vi "Assign X Coordinate.vi"(7 "Column Gap":i32=30, 10 "Order":T2[](array[typedef]), 11 "Decision Tree Out in":T1) -> (3 "Decision Tree Out out":T1)   [LabVIEW 2025]
uses:
  Types/Decision Tree.ctl
  Types/Sequencing Tree Node.ctl
  Types/Single Cmd Info.ctl
  <vilib>/picture/picture.llb/imagedata.ctl
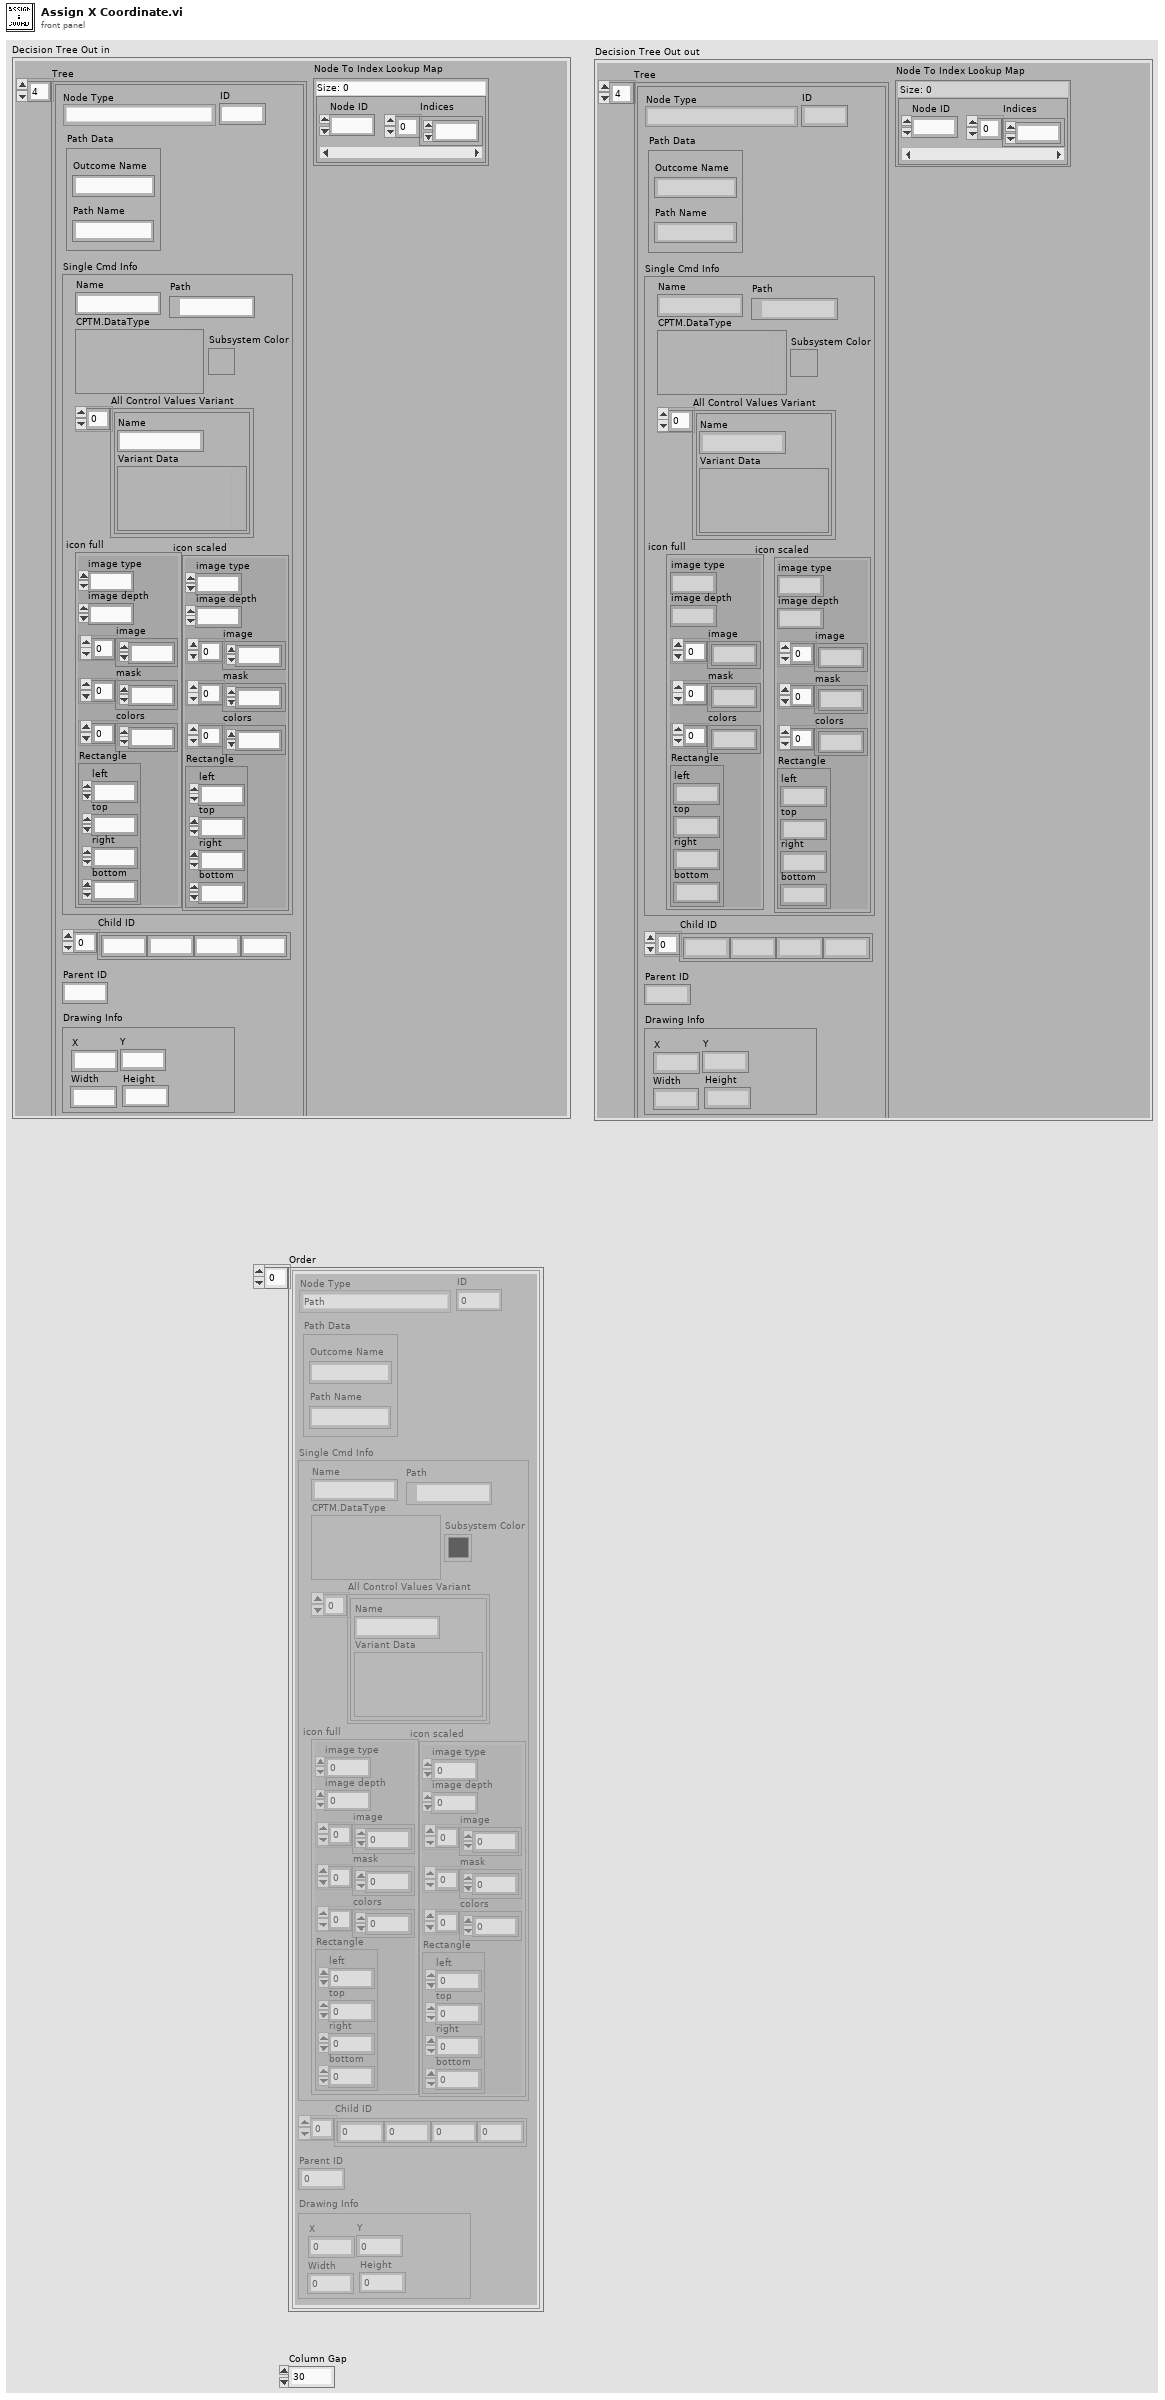
[diagram p1: front panel]
types:
  T1 = typedef "Decision Tree.ctl" = cluster{"Tree":T2[], "Node To Index Lookup Map":map{i16, i16[]}}
  T2 = typedef "Sequencing Tree Node.ctl" = cluster{"Node Type":enum16{"Path", "Command", "Leaf"}, "ID":i16, "Path Data":cluster{"Path Name":string, "Outcome Name":string}, "Single Cmd Info":T3, "Child ID":i32[], "Parent ID":i32, "Drawing Info":cluster{"X":i32, "Y":i32, "Width":i32, "Height":i32}}
  T3 = typedef "Single Cmd Info.ctl" = cluster{"Name":string, "CPTM.DataType":variant, "All Control Values Variant":cluster{"Name":string, "Variant Data":variant}[], "icon full":T4, "icon scaled":T4, "Path":path, "Subsystem Color":u32}
  T4 = typedef "imagedata.ctl" = cluster{"image type":i32, "image depth":i32, "image":u8[], "mask":u8[], "colors":u32[], "Rectangle":cluster{"left":i16, "top":i16, "right":i16, "bottom":i16}}
  T5 = cluster{"X":i32, "Y":i32, "Width":i32, "Height":i32}
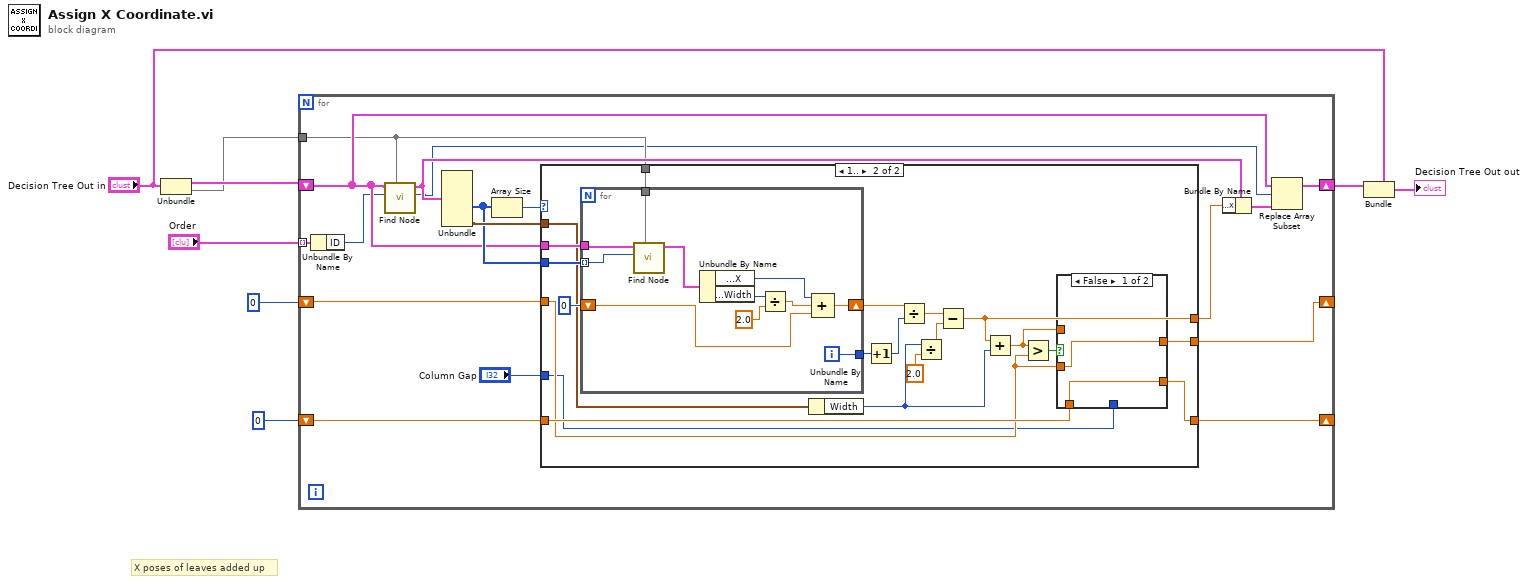
[diagram p0: block diagram]
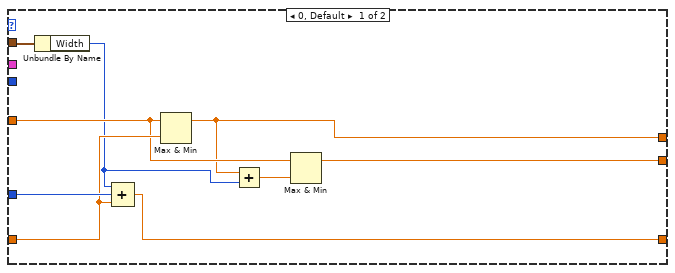
[diagram p2: hidden frame]
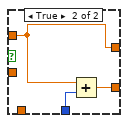
[diagram p3: hidden frame]
diagram:
  # "X poses of leaves added up"
  n1 = Unbundle("Decision Tree Out in") -> ("Tree"=w5:T2[], "Node To Index Lookup Map"=w1:map{i16, i16[]})
  n2 = for {
    tunnel: "Order" -> [w25] mode=indexing
    shift-right: [w19] -> _
    shift-left: 0 -> [w23]
    shift-right: [w16] -> w4
    shift-left: w5 -> [w13]
    shift-right: [w14] -> _
    shift-left: 0 -> [w15]
    tunnel: w1 -> [w10]
    n3 = Unbundle By Name(w25) -> ("ID"=w12:i16)
    n4 = call "Find Node.vi"("Node To Index Lookup Map"=w10, "ID"=w12, "Tree"=w13) -> ("Index"=w9:i16, "Node"=w11:T2)  [unwired: 7 in]
    n5 = Unbundle(w11) -> ("Child ID"=w18:i32[], "Drawing Info"=w20:T5)  [unwired: 5 out]
    n6 = Array Size(array=w18) -> (size(s)=w24:i32)
    n7 = case shown="1.." w24 {
      tunnel: w23 -> [w31 w40]
      tunnel: [w29 w44] -> w22
      tunnel: "Column Gap" -> [w32 w36]
      tunnel: w20 -> [w34 w45]
      tunnel: [w33 w39] -> w19
      tunnel: w18 -> [_ w54]
      tunnel: w13 -> [_ w53]
      tunnel: w15 -> [w30 w38]
      tunnel: [w26 w37] -> w14
      tunnel: w10 -> [_ w35]
      frame 0, Default {
        n8 = Unbundle By Name(w34) -> ("Width"=w28:i32)
        n9 = Compound Arithmetic op=ADD(w28, w32, w31) -> (w33:dbl)
        n10 = Max & Min(x=w30, y=w31) -> (max(x,y)=w29:dbl)  [unwired: 1 out]
        n11 = Add(x=w29, y=w28) -> (x+y=w27:dbl)
        n12 = Max & Min(x=w30, y=w27) -> (max(x,y)=w26:dbl)  [unwired: 1 out]
      }
      frame 1.. {
        n13 = for {
          tunnel: w54 -> [w61] mode=indexing
          tunnel: w53 -> [w62]
          shift-right: [w65] -> w51
          shift-left: 0 -> [w66]
          tunnel: [w64] -> w50
          tunnel: w35 -> [w60]
          i -> [w64]
          n14 = call "Find Node.vi"("Node To Index Lookup Map"=w60, "ID"=w61, "Tree"=w62) -> ("Node"=w63:T2)  [unwired: 7 in, 1 out]
          n15 = Unbundle By Name(w63) -> ("Drawing Info.X"=w68:i32, "Drawing Info.Width"=w70:i32)
          n16 = Divide(x=w70, y=2.0) -> (x/y=w67:dbl)
          n17 = Compound Arithmetic op=ADD(w68, w67, w66) -> (w65:dbl)
        }
        n18 = Unbundle By Name(w45) -> ("Width"=w43:i32)
        n19 = Increment(x=w50) -> (x+1=w49:i32)
        n20 = Divide(x=w51, y=w49) -> (x/y=w48:dbl)
        n21 = Divide(x=w43, y=2.0) -> (x/y=w47:dbl)
        n22 = Subtract(x=w48, y=w47) -> (x-y=w44:dbl)
        n23 = Add(x=w44, y=w43) -> (x+y=w41:dbl)
        n24 = Greater?(x=w41, y=w38) -> (0:w42:bool)
        n25 = case shown="False" w42 {
          tunnel: w41 -> [_ w58]
          tunnel: w40 -> [w56 _]
          tunnel: [w56 w59] -> w39
          tunnel: w38 -> [w55 _]
          tunnel: [w55 w58] -> w37
          tunnel: w36 -> [_ w57]
          frame False {
          }
          frame True {
            n26 = Add(x=w58, y=w57) -> (x+y=w59:dbl)
          }
        }
      }
    }
    n27 = Bundle By Name(cluster=w11, "Drawing Info.X"=w22) -> (w17:T2)
    n28 = Replace Array Subset(array=w13, new element=w17, index=w9) -> (w16:T2[])
  }
  n29 = Bundle(cluster="Decision Tree Out in", "Tree"=w4) -> (→"Decision Tree Out out":T1)  [unwired: 1 in]
